vi "UDP Sender generic_2.vi"(1 "re-initialise":bool, 2 "Show panel":bool, 3 "Spots":T4[](array[typedef])=[{"Position"={"x"=6.0125e-05, "y"=5.4187499999999996e-05, "z"=7.0069138e-06}, "Intensity"=1.0, "Vortex Charge"=0, "Phase"=1.0, "NA Position"={"x"=0.0, "y"=0.0, "r"=1.0}, "Line Trapping"={"Vector"={"x"=0.0, "y"=0.0, "z"=0.0}, "Phase Gradient"=0.0}, "Amplitude Correction"=0.0}, {"Position"={"x"=5.4116381799999997e-05, "y"=3.98060334e-05, "z"=0.0}, "Intensity"=1.0, "Vortex Charge"=0, "Phase"=1.0, "NA Position"={"x"=0.0, "y"=0.0, "r"=1.0}, "Line Trapping"={"Vector"={"x"=0.0, "y"=0.0, "z"=0.0}, "Phase Gradient"=0.0}, "Amplitude Correction"=0.0}, {"Position"={"x"=7.662499999999999e-05, "y"=4.6e-05, "z"=0.0}, "Intensity"=1.0, "Vortex Charge"=0, "Phase"=1.0, "NA Position"={"x"=0.0, "y"=0.0, "r"=1.0}, "Line Trapping"={"Vector"={"x"=0.0, "y"=0.0, "z"=0.0}, "Phase Gradient"=0.0}, "Amplitude Correction"=0.0}] {"Amplitude Correction" step=0.1; "Line Trapping"."Phase Gradient" step=0.05; "Line Trapping"."Vector"."x" step=1e-06 format="%#_6p"; "Line Trapping"."Vector"."y" step=1e-06 format="%#_6p"; "Line Trapping"."Vector"."z" step=1e-06 format="%#_6p"; "NA Position"."r" step=1e-06; "NA Position"."y" step=1e-06; "NA Position"."x" step=1e-06; "Position"."z" step=1e-06; "Position"."y" step=1e-06; "Position"."x" step=1e-06; "Phase" step=0.7753; "Intensity" step=0.1}) -> (0 "length":i32=557)   [LabVIEW 2010]
doc: "This VI sends UDP packets to the hologram server so that it can display holograms. It also has a lot of settings on the front panel, which control most of the aspects of hologram generation and display.\n\n\n(the line below ensures settings are saved)\n[Red Tweezers Save Settings]"
uses:
  spot.ctl
  line_trapping.ctl
  red_tweezers_globals_INTERNAL.vi
  <vilib>/Analysis/7linalg.llb/Create Special Real Matrix.vi
  <vilib>/Analysis/baseanly.llb/Real A x B.vi
  <vilib>/Analysis/NI_AALPro.lvlib
  <vilib>/Analysis/NI_AALBase.lvlib
panel:
  in  "SLM Settings":T1(tab)=enum."Output Location"
  out "LUT":cluster{dbl, dbl}[](graph)=[{-3.141592653589793, 0.0}, {-2.938909256584, 0.0}, {-2.736225859578207, 0.0}, {-2.533542462572414, 0.0}, {-2.330859065566621, 0.0}, {-2.1281756685608277, 0.0}, {-1.9254922715550344, 0.0}, {-1.7228088745492414, 0.0}, {-1.5201254775434483, 0.0}, {-1.317442080537655, 0.0}, {-1.114758683531862, 0.013893883492187394}, {-0.9120752865260688, 0.08758036091961133}, {-0.7093918895202758, 0.17634603660070491}, {-0.5067084925144827, 0.2746032303815977}, {-0.3040250955086896, 0.37671834381730007}, {-0.10134169850289654, 0.4770577784628228}, {0.10134169850289654, 0.5700419053299409}, {0.30402509550868917, 0.6525515168106174}, {0.5067084925144831, 0.7248906022855592}, {0.7093918895202758, 0.7876162829469834}, {0.9120752865260693, 0.8412856799871068}, {1.1147586835318615, 0.8864559145981461}, {1.3174420805376554, 0.9236841079723185}, {1.5201254775434485, 0.9535273813018404}, {1.7228088745492416, 0.9765739527614036}, {1.9254922715550338, 0.993632504666451}, {2.1281756685608277, 1.0}, {2.330859065566621, 1.0}, {2.533542462572414, 1.0}, {2.736225859578207, 1.0}, {2.938909256584, 1.0}, {3.141592653589793, 1.0}]
  in  "LUT File":path=path "C:/Users/alinnenberger/Desktop/Cube/red_tweezers_1_4_rc0/slm2040.LUT"
  in  "Intensity Masking (0=off, 1=on, >1=partially on)":dbl
  in  "Full Screen":bool
  out "Monitor Picture":picture
  in  "Monitor":i32=1
  in  "Zernike Coefficients":dbl[](array[numeric])=[0.0, 20.0, 20.0, 0.0, 0.0, 0.0, 0.0, 0.0, 0.0, 0.0, 0.0, 0.0]
  in  "Enable":bool=TRUE
  in  "Multiplier":dbl=1.0
  out "Phase Map":dbl[][](graph)
  in  "Physical Geometry":T2={"Hologram Size"={"x"=0.0102, "y"=0.0102}, "Focal Length"=0.0045, "Wavelength"=1.064e-06} {"Hologram Size"."y" min=0.0 max=1.0 step=0.001 format="%#_3p"; "Hologram Size"."x" min=0.0 max=1.0 step=0.001 format="%#_3p"; "Focal Length" format="%#_3p"; "Wavelength" format="%#_6p"}
  in  "Zero Position On Camera/pixels":cluster{"X":dbl, "Y":dbl}={"X"=320.0, "Y"=240.0}
  in  "Camera Pixel Size/m":cluster{dbl, dbl}={1e-07, 1e-07} {"?" format="%#_4p"; "?" format="%#_4p"}
  in  "Illumination Centre (range: 0 to 1)":cluster{"x":dbl, "y":dbl}={"x"=0.5, "y"=0.5} {"y" min=0.0 max=1.0 step=0.001; "x" min=0.0 max=1.0 step=0.001}
  in  "Scale Spot Positions":cluster{"x":dbl, "y":dbl, "z":dbl}={"x"=1.0, "y"=1.0, "z"=1.0} {"z" step=0.05 format="%#_3p"; "y" step=0.05 format="%#_3p"; "x" step=0.05 format="%#_3p"}
  in  "Rotation (degrees)":dbl
  in  "Tab Control":T3(tab)
  out "message":string="<data>\n<uniform id=0>\n  3.000000\r\n</uniform>\n<uniform id=2>\n  60.125000 54.187500 7.006914 0.000000 1.000000 1.000000 0.000000 0.000000 0.000000 0.000000 1.000000 0.000000 0.000000 0.000000 0.000000 0.000000 54.116382 39.806033 0.000000 0.000000 1.000000 1.000000 0.000000 0.000000 0.000000 0.000000 1.000000 0.000000 0.000000 0.000000 0.000000 0.000000 76.625000 46.000000 0.000000 0.000000 1.000000 1.000000 0.000000 0.000000 0.000000 0.000000 1.000000 0.000000 0.000000 0.000000 0.000000 0.000000\r\n</uniform>\n<uniform id=1>\n  0.000000\r\n</uniform>\n</data>"
  in  "x":dbl[](array[numeric])=[0.0, 0.0, 0.0]
  in  "y":dbl[](array[numeric])=[0.0, 0.0, 0.0]
  in  "z":dbl[](array[numeric])=[0.0, 0.0, 0.0]
  in  "close":bool
  # "Look-Up Table\nThis curve controls the output level (0=black, 1=white) for a given phase on the SLM.  It can be used to optimise the hologram to direct as much light as possible into the first diffraction order, and is particularly useful when the SLM has a range of more or less than one wavelength."
  # "Intensity masking can modulate the LUT to shape intensity on the SLM.  Leave at 0 for most purposes."
  # "Find the SLM Monitor\nSelect the monitor that corresponds to the SLM.  Usually this will be the second monitor (i.e. number 2).  If you are using a BNS SLM, leave \"full screen\" unchecked; for Holoeye/Hamamatsu, push that button.\n\nThe box below shows the monitors attached to your computer, and a red box where the SLM window will appear.  The monitor numbers should be the same as those in the Windows monitor settings.  You can also click monitors below to select them."
  # "Aberration Correction\nThe engine allows Zernike polynomials to be added to the hologram to compensate for aberrations.  The coefficients can be adjusted here.  The polynomials included are the first 15, ignoring piston and tilt (as these are adjusted for each spot)."
  # "Scaling Factors\nYou should enter the dimensions of your system in the \"physical geometry\" box to set approximate scaling; the hologram size is the SLM size (normally square, as only the central square is used) AFTER any magnification when it's re-imaged, and the focal length is that of the objective lens.\n\nHere, you can also set the size of pixels on the camera (best done using a calibration slide) and the location of the zero order from the SLM.\n\nFine-tuning can be done on the \"Alignment & Centering\" tab."
  # "Centering\nIf the illumination of the SLM is off-centre, moving a spot in Z will also affect its position in X and Y (think of an off-centre lens).  The \"illumination centre\" can correct for this.  Setting this parameter correctly is particularly important if Laguerre-Gauss beams are to be used (i.e. spots with L not equal to 0).  The real centre of the hologram is at 0.5,0.5.  NB if this value is far from 0.5, 0.5 the system probably needs to be realigned."
  # "Scaling and Rotation\nThe scaling rand rotation controls allow you to compensate for the camera and SLM being rotated relative to each other, or for small variations from the geometrically predicted scale.  The scaling factors ought to be aroud unity.  Negative scaling factors will invert the corresponding axis.\nNB: Make sure the correct values are entered in the \"geometry\" tab first!"
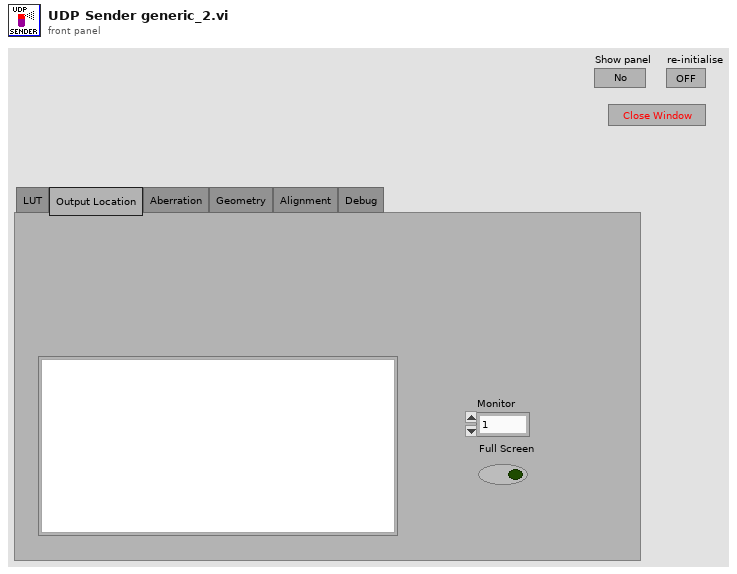
[diagram p1: front panel]
types:
  T1 = enum32{"LUT", "Output Location", "Aberration", "Geometry", "Alignment", "Debug"}
  T2 = cluster{"Hologram Size":cluster{"x":dbl, "y":dbl}, "Focal Length":dbl, "Wavelength":dbl}
  T3 = enum32{"Spots", "UDP Packets", "Field Tilt/Varying Astigmatism"}
  T4 = typedef "spot.ctl" = cluster{"Position":cluster{"x":dbl, "y":dbl, "z":dbl}, "Intensity":dbl, "Vortex Charge":i8, "Phase":dbl, "NA Position":cluster{"x":dbl, "y":dbl, "r":dbl}, "Line Trapping":T5, "Amplitude Correction":dbl}
  T5 = typedef "line_trapping.ctl" = cluster{"Vector":cluster{"x":dbl, "y":dbl, "z":dbl}, "Phase Gradient":dbl}
  T6 = enum32{"Identity", "Diagonal", "Toepliz", "Vandermonde", "Companion"}
  T7 = typedef "NI_Matrix.lvlib/RealMatrix.ctl" = dbl[][]
  T8 = typedef "LVMouseTypeDef.ctl" = cluster{"Mouse Position":cluster{"X":i32, "Y":i32}, "Mouse Modifiers":cluster{"Button Down":bool, "Shift Mod":bool, "Menu Mod":bool, "Option Mod":bool}}
  T9 = typedef "LVCursorListTypeDef.ctl" = cluster{"Name":string, "Color":u32, "Style":u8, "Point Style":u8, "Name Visible":bool, "Allow Drag":bool, "Cursor Mode":u32, "Plot":i32, "Index":i32, "Position":cluster{"X":dbl, "Y":dbl}, "X Scale":u32, "Y Scale":u32, "Watch Plots":i32[], "Watch All Plots":bool, "Plot Area":i32, "Label Offset":cluster{"X":dbl, "Y":dbl}}[]
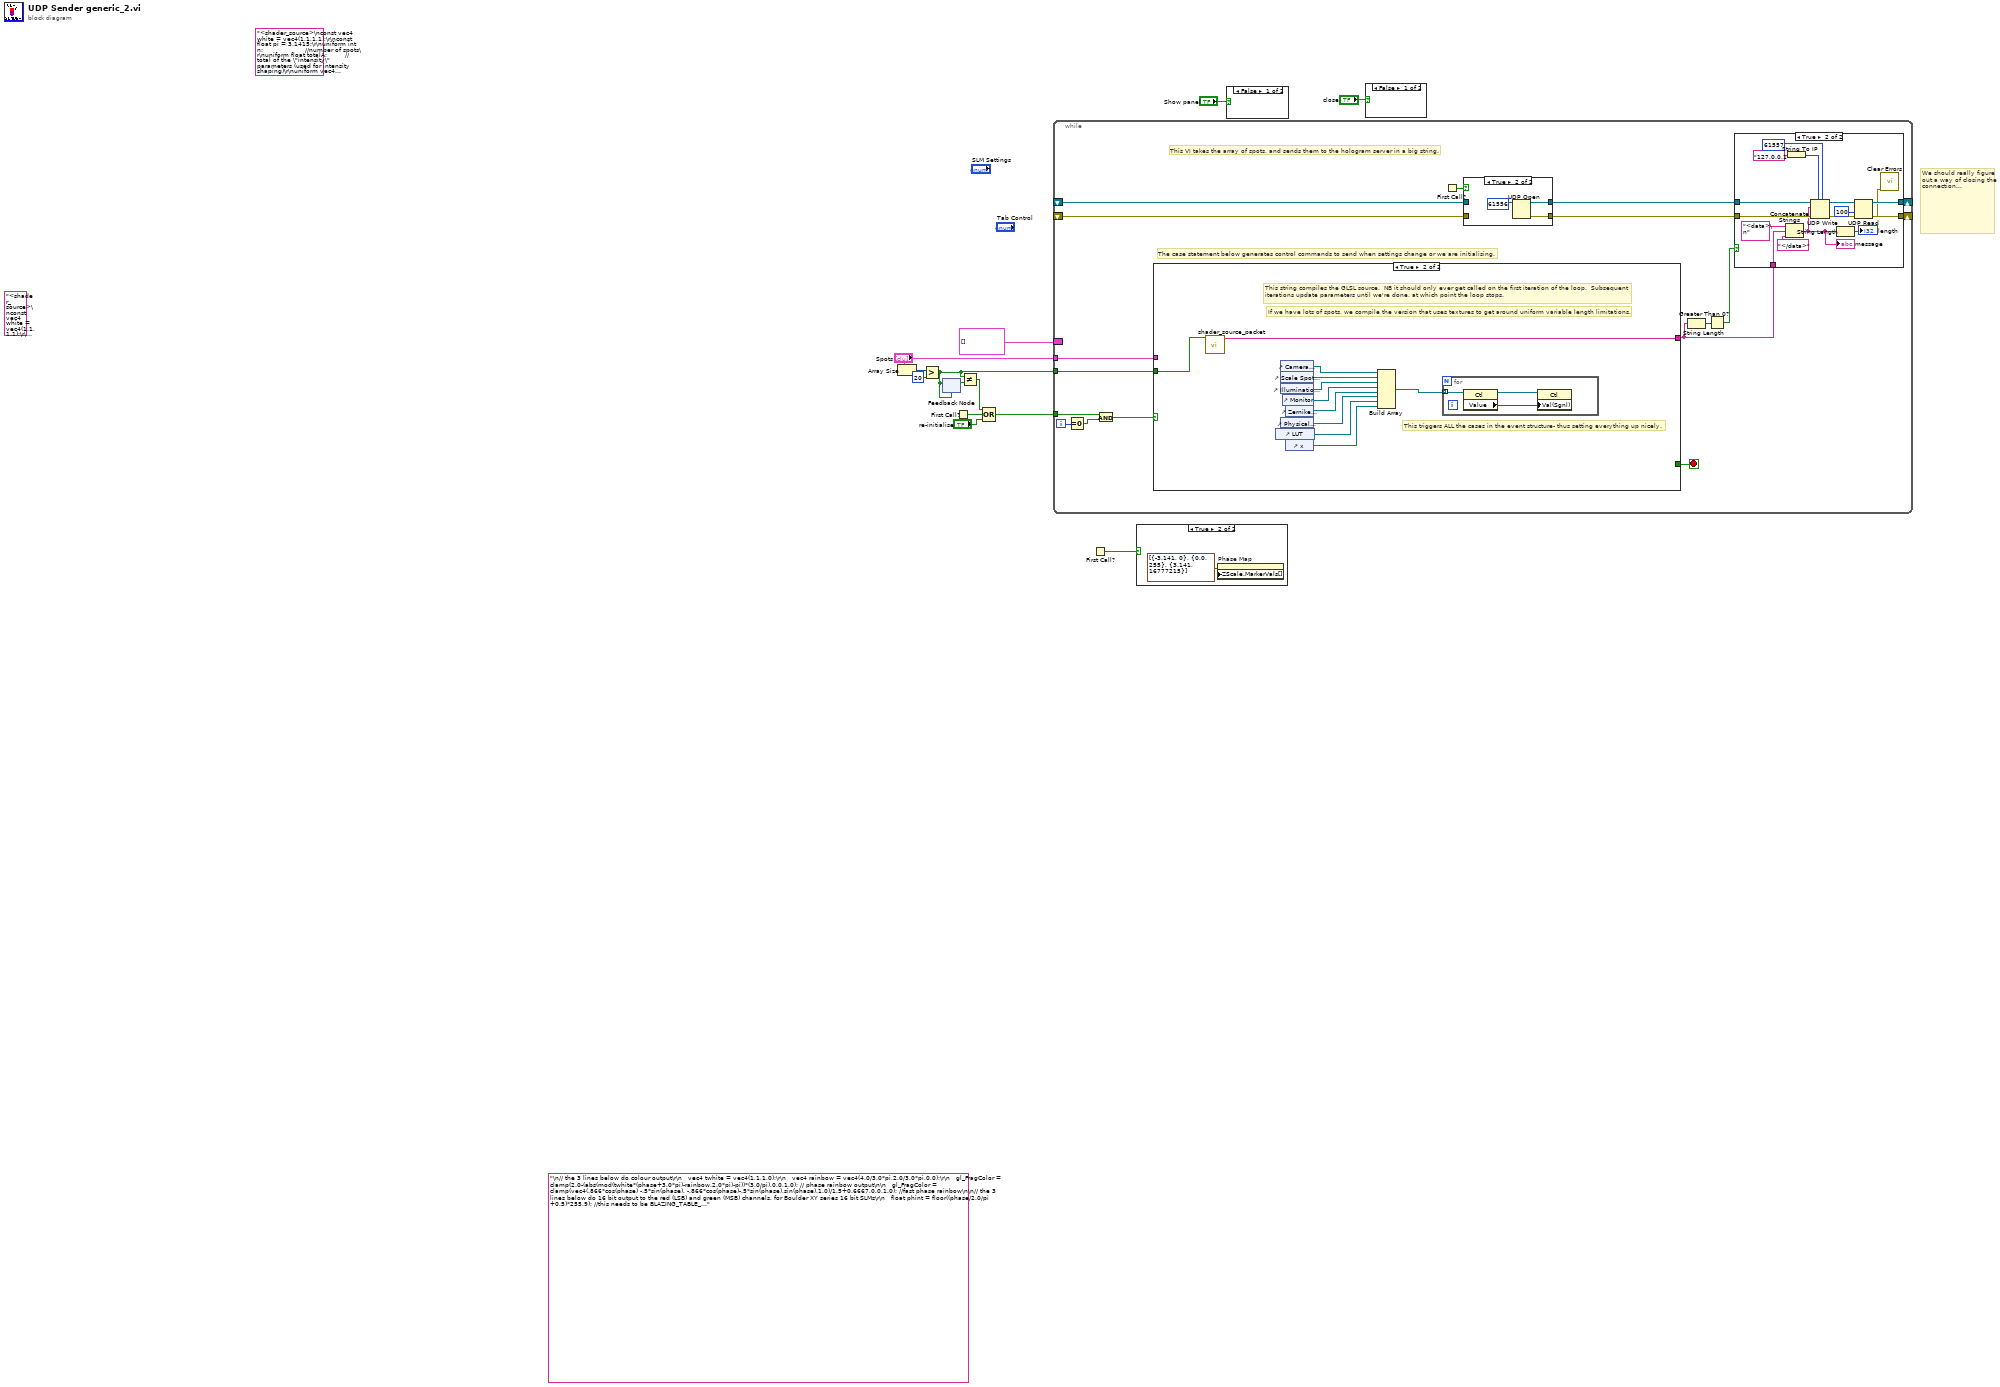
[diagram p0: block diagram]
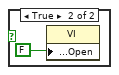
[diagram p3: hidden frame]
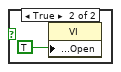
[diagram p4: hidden frame]
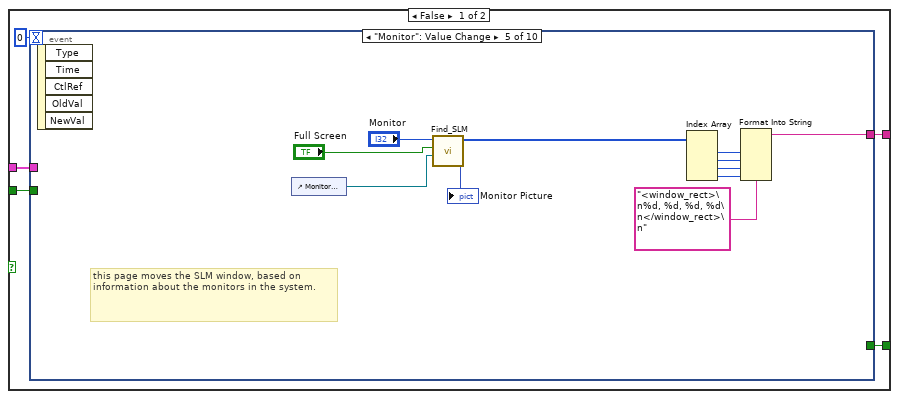
[diagram p6: hidden frame]
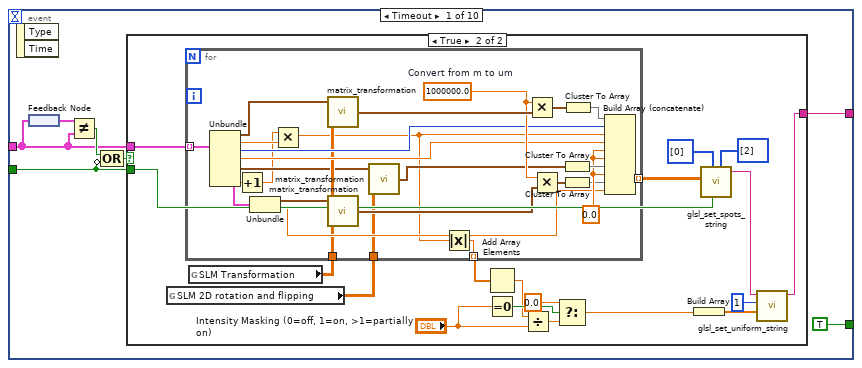
[diagram p7: hidden frame]
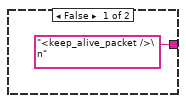
[diagram p8: hidden frame]
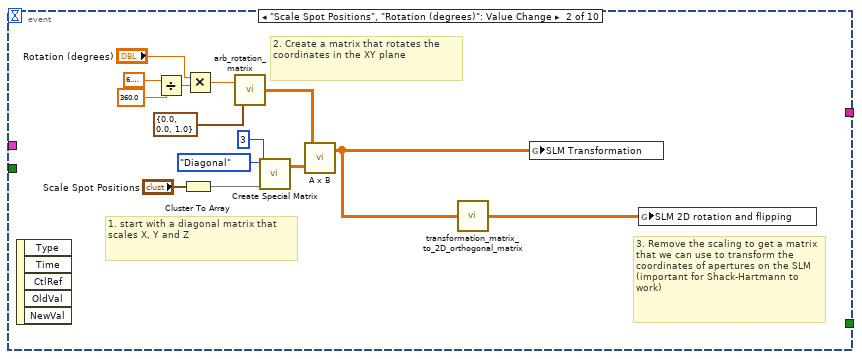
[diagram p9: hidden frame]
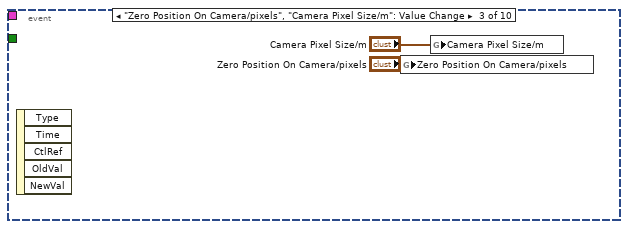
[diagram p10: hidden frame]
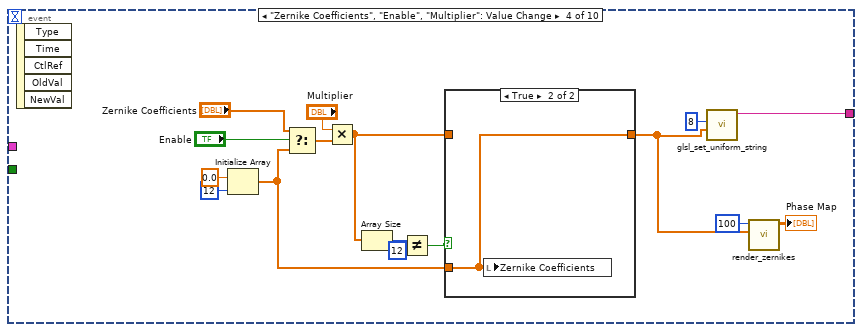
[diagram p11: hidden frame]
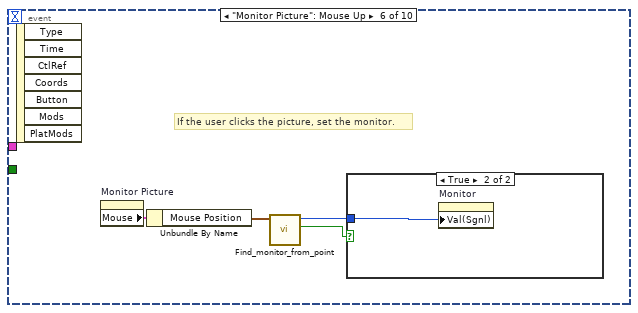
[diagram p13: hidden frame]
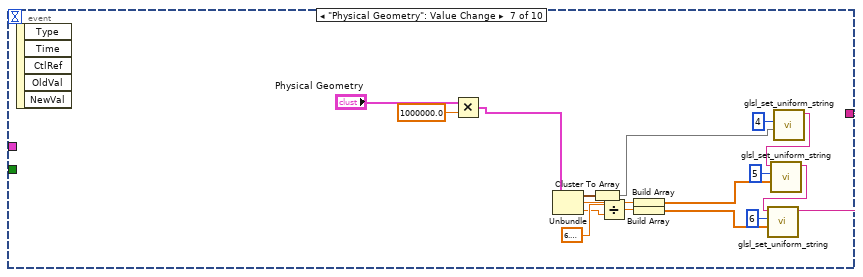
[diagram p15: hidden frame]
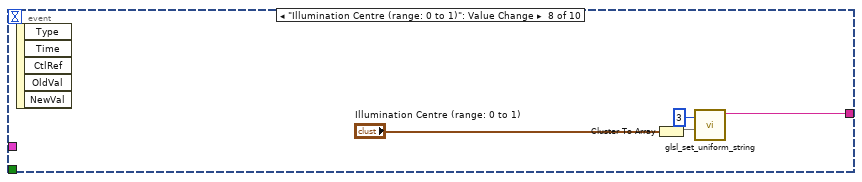
[diagram p16: hidden frame]
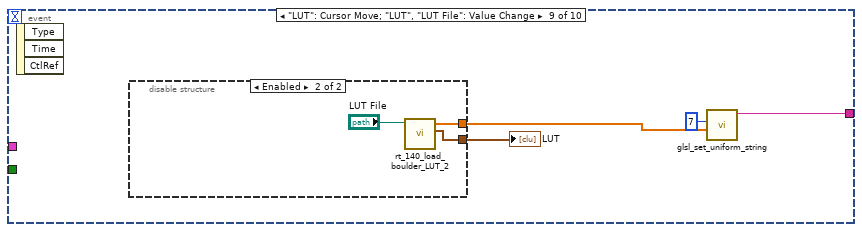
[diagram p17: hidden frame]
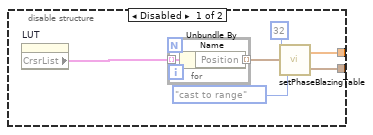
[diagram p18: hidden frame]
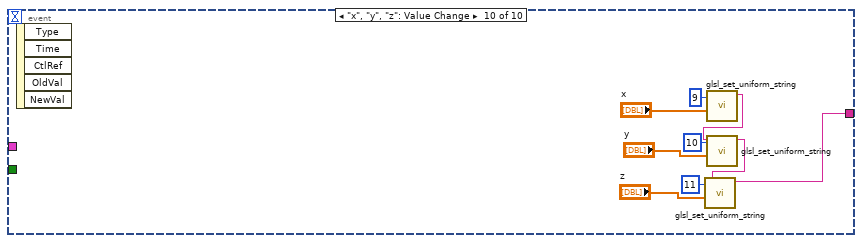
[diagram p19: hidden frame]
diagram:
  (unwired) "<shader_source>\nconst vec4 white = vec4(1,1,1,1);\r\nconst float pi = 3.1415;\r\nuniform int n;                     //number of spots\r\nuniform float totalA;         //total of the \"intensity\" parameters (used for intensity shaping)\r\nuniform sampler2D spots; //spot parameters- each spot corresponds to 4 vec4, first one is x,y,z,l, second one is amplitude, -,-,-\n\r                                            //element 0 x  y  z  l    (x,y,z in um and l is an integer)\n                                            //element 1 intensity (I) phase -  -\n                                            //element 2 na.x na.y na.r -  (the x, y position, and radius, of the spot on the SLM- useful for Shack-Hartmann holograms)\n                                            //element 3 line trapping x y z and phase gradient.  xyz define the size and angle of the line, phase gradient (between +/-1) is the\n                                            //scattering force component along the line.  Zero is usually a good choice for in-plane line traps\nuniform vec2 centre;        //=vec2(0.5,0.5);//centre of the hologram as a fraction of its size (usually 0.5,0.5)\r\nuniform vec2 size;            //=vec2(7000,7000);//size of the hologram in microns\r\nuniform float f;                 //=1600; //focal length in microns\r\nuniform float k;                //=9.36; //wavevector in 1/microns\r\nuniform float blazing[32]; //blazing function\r\nuniform vec4 zernikeCoefficients[3]; //zernike coefficients, matching the modes defined below\nuniform vec3 zernx;        //=vec3(0.0,0.0,0.0);\nuniform vec3 zerny;        //=vec3(0.0,0.0,0.0);\nuniform vec3 zernz;        //=vec3(0.0,0.0,0.0);\n\nvec4 spot(int i, int j){\n  return texture(spots, vec2( (float(j) +0.5) / 4.0, ( float(i) + 0.5) / float(n) ))*500.0 -250.0;\n}\n\nvoid main(void)\r\n{\n   float totalr=0.0;                                                //real and imaginary parts of the complex hologram for this pixel\r\n   float totali=0.0;\r\n   float phase;                                                       //phase of current pixel, due to the spot (in loop) or of the resultant hologram (after loop)\r\n   float amplitude;                                               //ditto for amplitude\r\n   vec2 xy=(gl_TexCoord[0].xy-centre)*size;    //current xy position in the hologram, in microns\r\n   float phi=atan(xy.x,xy.y);\t\t                              //angle of the line joining our point to the centre of the pattern\r\n   float length;                                                     //length of a line\r\n   vec4 pos=vec4(xy/f,1.0-dot(xy,xy)/2.0/f/f,phi/k);\r\n   vec4 na;                                                           //to be used later, inside the loop\r\n\t float sx;\r\n//Zernike polynomials\r\n   float x=xy.x/size.x*2.0;\n   float  y=xy.y/size.y*2.0; //x,y range from -1 to 1, because the Zernike modes want them to do that...\r\n   float r2=x*x+y*y;\r\n   vec4 zerna=vec4(2.0*x*y,2.0*r2-1.0,x*x-y*y,3.0*x*x*y-y*y*y); //zernike modes (2 -2, 2 0, 2 2, 3 -3)\r\n   vec4 zernb=vec4((3.0*r2-2.0)*y,(3.0*r2-2.0)*x,x*x*x-3.0*x*y*y,4.0*x*y*(x*x-y*y)); //3 -1 through 4 -4\r\n   vec4 zernc=vec4((4.0*r2-3.0)*zerna[0],6.0*r2*r2-6*r2+1,(4.0*r2-3.0)*zerna[2],x*x*x*x-6.0*x*x*y*y+y*y*y*y); //4 -2 through 4 4\r\n//probably want to redefine x,y,r2 if they are used below this line, but the are currently not.\n\n   vec4 varyingzernike=vec4(0.0,0.0,0.0,0.0);\n   varyingzernike.x=dot(zernx,zerna.xyz);\n   varyingzernike.y=dot(zerny,zerna.xyz);\n   varyingzernike.z=dot(zernz,zerna.xyz);\n\n   float j=0.0;                                                       //this loop goes through the spots and calculates the contribution from each one, summing\n                                                                            //real and imaginary parts as we go.\r\n   for(int i=0; i<n; i++){\n      amplitude=spot(i,1)[0];                             //amplitude of current spot\r\n      phase=k*dot(spot(i,0),pos)+spot(i,1)[1]; \n                                                                            //this is the basic gratings and lenses algorithm; phase=kx*x+ky*y+kz*(x^2+y^2)+l*theta\n\n      na = spot(i,2);                                           //restrict the spot to a region of the back aperture which is na[2] in radius, centred on na.xy\r\n      if(dot(na.xy-xy/size,na.xy-xy/size) > na[2]*na[2]){\n        amplitude = 0.0;\n      }\n//creates an xyz line trap, needs amplitude shaping.\n\r      vec4 line = spot(i,3);\n      length=sqrt(dot(line.xyz,line.xyz));\r\n      if(length>0.0){\r\n\t\t      sx=k*dot(vec4(pos.xyz,1.0*length),line);\r\n\t\t      if(sx!=0.0) amplitude*=sin(sx)/sx;\r\n      }\n\r                                                                 //finally, convert from amplitude+phase to real+imaginary for the summation\n      totalr += amplitude*sin(phase);\t  //the way atan is defined, we need to use sin for r and cos for i.\r\n      totali += amplitude*cos(phase);\r\n   }\n\r\n   amplitude = sqrt(totalr*totalr+totali*totali);\r\n   phase=atan(totalr,totali);\r\n   if(amplitude==0.0) phase=0.0;\r\n   if(totalA>0.0){ //do amplitude-shaping (dumps light into zero order when not needed)\r\n     phase *= clamp(amplitude/totalA,0.0,1.0);\r\n   }\r\n   phase += dot(zernikeCoefficients[0],zerna) + dot(zernikeCoefficients[1],zernb) + dot(zernikeCoefficients[2],zernc);\r\n   phase = mod(phase + pi, 2*pi) -pi;\n\r\n\n// the 3 lines below do blazed black and white output to all 3 colour channels (most SLMs use this)\n    //we split phase into two parts: phint is an integer between 0 and 30, alpha is a float between 0 and 0.99999999999999\n    //such that (phint + alpha)/31 maps onto 0...1.\n\r    //then we use the blazing array with linear interpolation to apply the LUT.\n\n   int phint = int(floor((phase/2.0/pi +0.5)*30.9999999)); //this needs to be BLAZING_TABLE_LENGTH-(something small)-1\r\n   float alpha = fract((phase/2.0/pi +0.5)*30.9999999);\r\n   gl_FragColor = white * blazing[phint]*(1.0-alpha)+blazing[phint+1]*alpha; //this uses the blazing table with linear interpolation\n\n//  gl_FragColor = spot(0,1);\n//  gl_FragColor = vec4(%%randcol%%);\n// gl_FragColor = gl_FragColor * vec4(%%randcol%%);\n//  gl_FragColor = texture(spots, gl_TexCoord[0].xy)*500.0-250.0;\n}\n</shader_source>\n\n<swap_buffers_at_refresh_rate>\n0\n</swap_buffers_at_refresh_rate>\n</data>"
  (unwired) "<shader_source>\nconst vec4 white = vec4(1,1,1,1);\r\nconst float pi = 3.1415;\r\nuniform int n;                     //number of spots\r\nuniform float totalA;         //total of the \"intensity\" parameters (used for intensity shaping)\r\nuniform vec4 spots[200]; //spot parameters- each spot corresponds to 4 vec4, first one is x,y,z,l, second one is amplitude, -,-,-\n\r                                            //element 0 x  y  z  l    (x,y,z in um and l is an integer)\n                                            //element 1 intensity (I) phase -  -\n                                            //element 2 na.x na.y na.r -  (the x, y position, and radius, of the spot on the SLM- useful for Shack-Hartmann holograms)\n                                            //element 3 line trapping x y z and phase gradient.  xyz define the size and angle of the line, phase gradient (between +/-1) is the\n                                            //scattering force component along the line.  Zero is usually a good choice for in-plane line traps\nuniform vec2 centre;        //=vec2(0.5,0.5);//centre of the hologram as a fraction of its size (usually 0.5,0.5)\r\nuniform vec2 size;            //=vec2(7000,7000);//size of the hologram in microns\r\nuniform float f;                 //=1600; //focal length in microns\r\nuniform float k;                //=9.36; //wavevector in 1/microns\r\nuniform float blazing[32]; //blazing function\r\nuniform vec4 zernikeCoefficients[3]; //zernike coefficients, matching the modes defined below\nuniform vec3 zernx;        //=vec3(0.0,0.0,0.0);\nuniform vec3 zerny;        //=vec3(0.0,0.0,0.0);\nuniform vec3 zernz;        //=vec3(0.0,0.0,0.0);\n\nvec4 spot(int i, int j){\n//  return texture(spots, vec2( (float(j) +0.5) / 4.0, ( float(i) + 0.5) / float(n) ))*500.0 -250.0;\n  return spots[4*i +j];\n}\n\nvoid main(void)\r\n{\n   float totalr=0.0;                                                //real and imaginary parts of the complex hologram for this pixel\r\n   float totali=0.0;\r\n   float phase;                                                       //phase of current pixel, due to the spot (in loop) or of the resultant hologram (after loop)\r\n   float amplitude;                                               //ditto for amplitude\r\n   vec2 xy=(gl_TexCoord[0].xy-centre)*size;    //current xy position in the hologram, in microns\r\n   float phi=atan(xy.x,xy.y);\t\t                              //angle of the line joining our point to the centre of the pattern\r\n   float length;                                                     //length of a line\r\n   vec4 pos=vec4(xy/f,1.0-dot(xy,xy)/2.0/f/f,phi/k);\r\n   vec4 na;                                                           //to be used later, inside the loop\r\n\t float sx;\r\n//Zernike polynomials\r\n   float x=xy.x/size.x*2.0;\n   float  y=xy.y/size.y*2.0; //x,y range from -1 to 1, because the Zernike modes want them to do that...\r\n   float r2=x*x+y*y;\r\n   vec4 zerna=vec4(2.0*x*y,2.0*r2-1.0,x*x-y*y,3.0*x*x*y-y*y*y); //zernike modes (2 -2, 2 0, 2 2, 3 -3)\r\n   vec4 zernb=vec4((3.0*r2-2.0)*y,(3.0*r2-2.0)*x,x*x*x-3.0*x*y*y,4.0*x*y*(x*x-y*y)); //3 -1 through 4 -4\r\n   vec4 zernc=vec4((4.0*r2-3.0)*zerna[0],6.0*r2*r2-6*r2+1,(4.0*r2-3.0)*zerna[2],x*x*x*x-6.0*x*x*y*y+y*y*y*y); //4 -2 through 4 4\r\n//probably want to redefine x,y,r2 if they are used below this line, but the are currently not.\n\n   vec4 varyingzernike=vec4(0.0,0.0,0.0,0.0);\n   varyingzernike.x=dot(zernx,zerna.xyz);\n   varyingzernike.y=dot(zerny,zerna.xyz);\n   varyingzernike.z=dot(zernz,zerna.xyz);\n\n   float j=0.0;                                                       //this loop goes through the spots and calculates the contribution from each one, summing\n                                                                            //real and imaginary parts as we go.\r\n   for(int i=0; i<n; i++){\n      amplitude=spot(i,1)[0];                             //amplitude of current spot\r\n      phase=k*dot(spot(i,0),pos)+spot(i,1)[1]; \n                                                                            //this is the basic gratings and lenses algorithm; phase=kx*x+ky*y+kz*(x^2+y^2)+l*theta\n\n      na = spot(i,2);                                           //restrict the spot to a region of the back aperture which is na[2] in radius, centred on na.xy\r\n      if(dot(na.xy-xy/size,na.xy-xy/size) > na[2]*na[2]){\n        amplitude = 0.0;\n      }\n//creates an xyz line trap, needs amplitude shaping.\n\r      vec4 line = spot(i,3);\n      length=sqrt(dot(line.xyz,line.xyz));\r\n      if(length>0.0){\r\n\t\t      sx=k*dot(vec4(pos.xyz,1.0*length),line);\r\n\t\t      if(sx!=0.0) amplitude*=sin(sx)/sx;\r\n      }\n\r                                                                 //finally, convert from amplitude+phase to real+imaginary for the summation\n      totalr += amplitude*sin(phase);\t  //the way atan is defined, we need to use sin for r and cos for i.\r\n      totali += amplitude*cos(phase);\r\n   }\n\r\n   amplitude = sqrt(totalr*totalr+totali*totali);\r\n   phase=atan(totalr,totali);\r\n   if(amplitude==0.0) phase=0.0;\r\n   if(totalA>0.0){ //do amplitude-shaping (dumps light into zero order when not needed)\r\n     phase *= clamp(amplitude/totalA,0.0,1.0);\r\n   }\r\n   phase += dot(zernikeCoefficients[0],zerna) + dot(zernikeCoefficients[1],zernb) + dot(zernikeCoefficients[2],zernc);\r\n   phase = mod(phase + pi, 2*pi) -pi;\n\r\n\n// the 3 lines below do blazed black and white output to all 3 colour channels (most SLMs use this)\n    //we split phase into two parts: phint is an integer between 0 and 30, alpha is a float between 0 and 0.99999999999999\n    //such that (phint + alpha)/31 maps onto 0...1.\n\r    //then we use the blazing array with linear interpolation to apply the LUT.\n\n   int phint = int(floor((phase/2.0/pi +0.5)*30.9999999)); //this needs to be BLAZING_TABLE_LENGTH-(something small)-1\r\n   float alpha = fract((phase/2.0/pi +0.5)*30.9999999);\r\n   gl_FragColor = white * blazing[phint]*(1.0-alpha)+blazing[phint+1]*alpha; //this uses the blazing table with linear interpolation\n\n//  gl_FragColor = spot(0,1);\n//  gl_FragColor = vec4(%%randcol%%);\n// gl_FragColor = gl_FragColor * vec4(%%randcol%%);\n//  gl_FragColor = texture(spots, gl_TexCoord[0].xy)*500.0-250.0;\n}\n</shader_source>\n\n<swap_buffers_at_refresh_rate>\n0\n</swap_buffers_at_refresh_rate>\n</data>"
  (unwired) "\n// the 3 lines below do colour output\r\n   vec4 twhite = vec4(1,1,1,0);\r\n   vec4 rainbow = vec4(4.0/3.0*pi,2.0/3.0*pi,0,0);\r\n   gl_FragColor = clamp(2.0-(abs(mod(twhite*(phase+3.0*pi)-rainbow,2.0*pi)-pi))*(3.0/pi),0.0,1.0); // phase rainbow output\n\n   gl_FragColor = clamp(vec4(.866*cos(phase) -.5*sin(phase), -.866*cos(phase)-.5*sin(phase),sin(phase),1.0)/1.5+0.6667,0.0,1.0); //fast phase rainbow\n\n// the 3 lines below do 16 bit output to the red (LSB) and green (MSB) channels, for Boulder XY series 16 bit SLMs\r\n   float phint = floor((phase/2.0/pi +0.5)*255.9); //this needs to be BLAZING_TABLE_LENGTH-(something small)\r\n   float alpha = fract((phase/2.0/pi +0.5)*255.9);\r\n   gl_FragColor = vec4(alpha,phint/255.0,0.0,1.0); //this uses the blazing table with linear interpolation\r\n\n// This one does grayscale output, black=-pi white=pi\r\n   gl_FragColor = white*(phase/2.0/pi +0.5);\n\r\n// the 3 lines below do blazed black and white output to all 3 colour channels (most SLMs use this)\r\n   int phint = int(floor((phase/2.0/pi +0.5)*30.9999999)); //this needs to be BLAZING_TABLE_LENGTH-(something small)-1\r\n   float alpha = fract((phase/2.0/pi +0.5)*30.9999999);\r\n   gl_FragColor = white * blazing[phint]*(1.0-alpha)+blazing[phint+1]*alpha; //this uses the blazing table with linear interpolation\n\n// \t gl_FragColor = float(n)*spots[0][1]/4.0*white;\r\n// \t gl_FragColor = mod(y*5,1.0)*white;\n//   gl_FragColor = white*blazing[16];\n\r"
  # "We should really figure out a way of closing the connection..."
  n1 = Array Size(array="Spots") -> (size(s)=w6:i32)
  n2 = Greater?(x=w6, y=20) -> (0:w2:bool)
  n3 = feedback #1(w2) -> (w8:bool)
  n4 = feedback-in #1(w2) -> ()
  n5 = First Call?() -> (First Call?: T/F=w5:bool)
  n6 = Not Equal?(x=w2, y=w8) -> (x != y?=w9:bool)
  n7 = Compound Arithmetic op=OR(w9, w5, "re-initialise") -> (w4:bool)
  n8 = while {
    shift-right: [w29] -> _
    shift-left: _ -> [w28]
    shift-right: [w30] -> _
    shift-left: _ -> [w27]
    border: T4[] [] ("Spots 2") -> [_]
    tunnel: w4 -> [w19]
    tunnel: w2 -> [w18]
    tunnel: "Spots" -> [w14]
    i -> [w16]
    stop <- w23 stop-if-true
    # "The case statement below generates control commands to send when settings change or we are initialising."
    # "This VI takes the array of spots, and sends them to the hologram server in a big string."
    n9 = Equal To 0?(x=w16) -> (x = 0?=w15:bool)
    n10 = And(x=w19, y=w15) -> (x .and. y?=w17:bool)
    n11 = case shown="True" w17 {
      tunnel: [w51 w201] -> w22
      tunnel: [w50 _] -> w23
      tunnel: w14 -> [w49 _]
      tunnel: w18 -> [w48 w200]
      frame False {
        n12 = event shown="[4] \"Monitor\": Value Change" {
          selector: _ -> [_ _ _ _ _ _ _ _ _ _]
          dyn-events: _ -> [_ _ _ _ _ _ _ _ _ _]
          timeout: 0 -> [_ _ _ _ _ _ _ _ _ _]
          tunnel: [w59 _ _ w121 w140 _ w155 w172 w176 w191] -> w51
          tunnel: [TRUE _ _ _ _ _ _ _ _ _] -> w50
          tunnel: w49 -> [w55 _ _ _ _ _ _ _ _ _]
          tunnel: w48 -> [w54 _ _ _ _ _ _ _ _ _]
          event Timeout {
            n13 = event-data() -> ()  [unwired: 1 in, 2 out]
            n14 = feedback #2() -> (w56:T4[])
            n15 = feedback-in #2(w55) -> ()
            n16 = Not Equal?(x=w56, y=w55) -> (x != y?=w57:bool)
            n17 = Compound Arithmetic op=OR(w57, invert w54) -> (w53:bool)
            n18 = case shown="True" w53 {
              tunnel: ["<keep_alive_packet />\n" ("Uniform-setting string") w69] -> w59
              tunnel: w55 -> [_ w62]
              tunnel: w54 -> [_ w61]
              frame False {
              }
              frame True {
                n19 = global read "red_tweezers_globals_INTERNAL.vi" "SLM 2D rotation and flipping"() -> (w67:T7)
                n20 = global read "red_tweezers_globals_INTERNAL.vi" "SLM Transformation"() -> (w68:T7)
                n21 = for {
                  tunnel: w62 -> [w102] mode=indexing
                  tunnel: [w99] -> w70 mode=indexing
                  tunnel: [w95] -> w66 mode=indexing
                  tunnel: w68 -> [w86]
                  tunnel: w67 -> [w82]
                  w91 = 0.0 ("element")
                  w96 = 1000000.0  # Convert from m to um
                  n22 = Unbundle(w102) -> ("Position"=w87:cluster{"x":dbl, "y":dbl, "z":dbl}, "Intensity"=w93:dbl, "Vortex Charge"=w94:i8, "Phase"=w92:dbl, "NA Position"=w84:cluster{"x":dbl, "y":dbl, "r":dbl}, "Line Trapping"=w100:T5, "Amplitude Correction"=w80:dbl)
                  n23 = Increment(x=w80) -> (x+1=w79:dbl)
                  n24 = Unbundle(w100) -> ("Vector"=w88:cluster{"x":dbl, "y":dbl, "z":dbl}, "Phase Gradient"=w89:dbl)
                  n25 = Multiply(x=w79, y=w93) -> (x*y=w81:dbl)
                  n26 = call "matrix_transformation.vi"("Transformation Matrix"=w86, "Input Vector"=w87) -> ("Output Vector"=w104:cluster{dbl, dbl, dbl})  [unwired: 1 in, 1 out]
                  n27 = call "matrix_transformation.vi"("Transformation Matrix"=w86, "Input Vector"=w88) -> ("Output Vector"=w85:cluster{dbl, dbl, dbl})  [unwired: 1 in, 1 out]
                  n28 = call "matrix_transformation.vi"("Transformation Matrix"=w82, "Input Vector"=w84) -> ("Output Vector"=w83:cluster{dbl, dbl, dbl})  [unwired: 1 in, 1 out]
                  n29 = Absolute Value(x=w81) -> (abs(x)=w99:dbl)
                  n30 = Multiply(x=w96, y=w104) -> (x*y=w98:cluster{dbl, dbl, dbl})
                  n31 = Multiply(x=w96, y=w85) -> (x*y=w97:cluster{dbl, dbl, dbl})
                  n32 = Cluster To Array(cluster=w83) -> (array=w101:dbl[])
                  n33 = Cluster To Array(cluster=w97) -> (array=w90:dbl[])
                  n34 = Cluster To Array(cluster=w98) -> (array=w103:dbl[])
                  n35 = Build Array (concatenate)(w103, w94, w81, w92, w91, w91, w101, w91, w90, w89) -> (w95:dbl[])
                }
                n36 = Add Array Elements(numeric array=w70) -> (sum=w71:dbl)
                n37 = Equal To 0?(x="Intensity Masking (0=off, 1=on, >1=partially on)") -> (x = 0?=w74:bool)
                n38 = Divide(x=w71, y="Intensity Masking (0=off, 1=on, >1=partially on)") -> (x/y=w73:dbl)
                n39 = Select(t=0.0, s=w74, f=w73) -> (s? t:f=w77:dbl)
                n40 = Build Array(w77) -> (w78:dbl[])
                n41 = call "glsl_set_spots_string.vi"("spots uniforms"=i32[] [2], "Use Textures?"=w61, "n uniforms"=i32[] [0], "Spots (2D Array)"=w66) -> ("Uniform-Setting String"=w65:string)  [unwired: 7 in]
                n42 = call "glsl_set_uniform_string.vi"("Uniform Value"=w78, "uniform index"=1, "initial string"=w65) -> ("Uniform-setting string"=w69:string)  [unwired: 3 in, 1 out]
              }
            }
          }
          event "Scale Spot Positions", "Rotation (degrees)": Value Change {
            # "3. Remove the scaling to get a matrix that we can use to transform the coordinates of apertures on the SLM (important for Shack-Hartmann to work)"
            # "2. Create a matrix that rotates the coordinates in the XY plane"
            # "1. start with a diagonal matrix that scales X, Y and Z"
            n43 = event-data() -> ()  [unwired: 1 in, 5 out]
            n44 = Divide(x=6.283185307179586, y=360.0) -> (x/y=w110:dbl)
            n45 = Cluster To Array(cluster="Scale Spot Positions") -> (array=w115:dbl[])
            n46 = Multiply(x="Rotation (degrees)", y=w110) -> (x*y=w108:dbl)
            n47 = call "arb_rotation_matrix.vi"("Unit Vector"=cluster{dbl, dbl, dbl} {0.0, 0.0, 1.0}, "theta"=w108) -> ("Real Matrix"=w113:T7)
            n48 = call-poly <vilib>:"Create Special Matrix.vi"("matrix type"=T6."Diagonal", "matrix size"=3, "Input Vector1"=w115) -> ("Special Matrix"=w112:T7)  [unwired: 2 in, 1 out]
            n49 = call-poly <vilib>:"A x B.vi"("B"=w112, "A"=w113) -> ("A x B"=w106:T7)  [unwired: 1 out]
            n50 = call "transformation_matrix_to_2D_orthogonal_matrix.vi"("A x B"=w106) -> ("Real Matrix"=w105:T7)
            n51 = global write "red_tweezers_globals_INTERNAL.vi" "SLM Transformation"(w106) -> ()
            n52 = global write "red_tweezers_globals_INTERNAL.vi" "SLM 2D rotation and flipping"(w105) -> ()
          }
          event "Zero Position On Camera/pixels", "Camera Pixel Size/m": Value Change {
            n53 = event-data() -> ()  [unwired: 1 in, 5 out]
            n54 = global write "red_tweezers_globals_INTERNAL.vi" "Zero Position On Camera/pixels"("Zero Position On Camera/pixels") -> ()
            n55 = global write "red_tweezers_globals_INTERNAL.vi" "Camera Pixel Size/m"("Camera Pixel Size/m") -> ()
          }
          event "Zernike Coefficients", "Enable", "Multiplier": Value Change {
            n56 = event-data() -> ()  [unwired: 1 in, 5 out]
            n57 = Initialize Array(0.0 ("element"), 12 ("dimension size")) -> (w124:dbl[])
            n58 = Select(t="Zernike Coefficients", s="Enable", f=w124) -> (s? t:f=w131:dbl[])
            n59 = Multiply(x="Multiplier", y=w131) -> (x*y=w123:dbl[])
            n60 = Array Size(array=w123) -> (size(s)=w127:i32)
            n61 = Not Equal?(x=w127, y=12) -> (x != y?=w125:bool)
            n62 = case shown="True" w125 {
              tunnel: w124 -> [_ w138]
              tunnel: w123 -> [w137 _]
              tunnel: [w137 w138] -> w122
              frame False {
              }
              frame True {
                n63 = local write "Zernike Coefficients"(w138) -> ()
              }
            }
            n64 = call "glsl_set_uniform_string.vi"("Uniform Value"=w122, "uniform index"=8) -> ("Uniform-setting string"=w121:string)  [unwired: 4 in, 1 out]
            n65 = call "render_zernikes.vi"("Size"=100, "Coefficients"=w122) -> ("Phase Map"=→"Phase Map":dbl[][])  [unwired: 6 out]
          }
          event "Monitor": Value Change {
            # "this page moves the SLM window, based on information about the monitors in the system."
            n66 = event-data() -> ()  [unwired: 1 in, 5 out]
            n67 = control-ref of="Monitor Picture"() -> (w147:refnum<vi>)
            n68 = call "Find_SLM.vi"("Picture Control"=w147, "Full Screen"="Full Screen", "Monitor"="Monitor") -> ("Monitor Picture"=→"Monitor Picture":picture, "Window Rect"=w141:i16[])  [unwired: 5 in, 2 out]
            n69 = Index Array(array=w141) -> (element #1=w143:i16, element #2=w144:i16, element #3=w145:i16, element #4=w146:i16)  [unwired: 4 in]
            n70 = Format Into String(format string="<window_rect>\n%d, %d, %d, %d\n</window_rect>\n", w143, w144, w145, w146) -> (resulting string=w140:string)  [unwired: 2 in, 1 out]
          }
          event "Monitor Picture": Mouse Up {
            # "If the user clicks the picture, set the monitor."
            n71 = event-data() -> ()  [unwired: 1 in, 7 out]
            n72 = property on="Monitor Picture" class="Pict"() -> ("Mouse"=w153:T8)  [unwired: 2 in, 2 out]
            n73 = Unbundle By Name(w153) -> ("Mouse Position"=w152:cluster{"X":i32, "Y":i32})
            n74 = call "Find_monitor_from_point.vi"("Point"=w152) -> ("In Monitor"=w151:bool, "Monitor"=w150:i32)  [unwired: 9 in]
            n75 = case shown="True" w151 {
              tunnel: w150 -> [_ w154]
              frame False {
              }
              frame True {
                n76 = property on="Monitor" class="DigNum (strict)"("Val(Sgnl)"=w154) -> ()  [unwired: 2 in, 2 out]
              }
            }
          }
          event "Physical Geometry": Value Change {
            n77 = event-data() -> ()  [unwired: 1 in, 5 out]
            n78 = Multiply(x="Physical Geometry", y=1000000.0 ("Wavevector (2pi/wavelength)")) -> (x*y=w163:T2)
            n79 = Unbundle(w163) -> ("Hologram Size"=w164:cluster{"x":dbl, "y":dbl}, "Focal Length"=w167:dbl, "Wavelength"=w170:dbl)
            n80 = Cluster To Array(cluster=w164) -> (array=w165:dbl[])
            n81 = Divide(x=6.283185307179586, y=w170) -> (x/y=w169:dbl)
            n82 = Build Array(w167) -> (w166:dbl[])
            n83 = Build Array(w169) -> (w168:dbl[])
            n84 = call "glsl_set_uniform_string.vi"("Uniform Value"=w165, "uniform index"=4) -> ("Uniform-setting string"=w157:string)  [unwired: 4 in, 1 out]
            n85 = call "glsl_set_uniform_string.vi"("Uniform Value"=w166, "uniform index"=5, "initial string"=w157) -> ("Uniform-setting string"=w156:string)  [unwired: 3 in, 1 out]
            n86 = call "glsl_set_uniform_string.vi"("Uniform Value"=w168, "uniform index"=6, "initial string"=w156) -> ("Uniform-setting string"=w155:string)  [unwired: 3 in, 1 out]
          }
          event "Illumination Centre (range: 0 to 1)": Value Change {
            n87 = event-data() -> ()  [unwired: 1 in, 5 out]
            n88 = Cluster To Array(cluster="Illumination Centre (range: 0 to 1)") -> (array=w174:dbl[])
            n89 = call "glsl_set_uniform_string.vi"("Uniform Value"=w174, "uniform index"=3) -> ("Uniform-setting string"=w172:string)  [unwired: 4 in, 1 out]
          }
          event "LUT": Cursor Move; "LUT", "LUT File": Value Change {
            n90 = event-data() -> ()  [unwired: 1 in, 3 out]
            n91 = disable-structure shown="Enabled" {
              disable-tunnel: [w185 w190] -> w178
              disable-tunnel: [w181 w189] -> w177
              frame Disabled {
                n92 = property on="LUT" class="XYGraph (strict)"() -> ("CrsrList"=w180:T9)  [unwired: 2 in, 2 out]
                n93 = for {
                  tunnel: w180 -> [w187] mode=indexing
                  tunnel: [w186] -> w184 mode=indexing
                  n94 = Unbundle By Name(w187) -> ("Position"=w186:cluster{"X":dbl, "Y":dbl})
                }
                n95 = call "setPhaseBlazingTable.vi"("-¹..¹ range control"=enum16{"wrap round", "cast to range"}."cast to range", "Anchor Points"=w184, "#elements (default 256)"=32) -> ("blazing graph"=w181:cluster{dbl, dbl}[], "blazing table"=w185:dbl[])
              }
              frame Enabled {
                n96 = call "rt_140_load_boulder_LUT_2.vi"("LUT File"="LUT File") -> ("'blazing function'"=w189:cluster{"X":dbl, "Y":dbl}[], "blazing table"=w190:dbl[])  [unwired: 8 in, 1 out]
              }
            }
            "LUT" <- w177
            n97 = call "glsl_set_uniform_string.vi"("Uniform Value"=w178, "uniform index"=7) -> ("Uniform-setting string"=w176:string)  [unwired: 4 in, 1 out]
          }
          event "x", "y", "z": Value Change {
            n98 = event-data() -> ()  [unwired: 1 in, 5 out]
            n99 = call "glsl_set_uniform_string.vi"("Uniform Value"="x", "uniform index"=9) -> ("Uniform-setting string"=w195:string)  [unwired: 4 in, 1 out]
            n100 = call "glsl_set_uniform_string.vi"("Uniform Value"="y", "uniform index"=10, "initial string"=w195) -> ("Uniform-setting string"=w196:string)  [unwired: 3 in, 1 out]
            n101 = call "glsl_set_uniform_string.vi"("Uniform Value"="z", "uniform index"=11, "initial string"=w196) -> ("Uniform-setting string"=w191:string)  [unwired: 3 in, 1 out]
          }
        }
      }
      frame True {
        # "If we have lots of spots, we compile the version that uses textures to get around uniform variable length limitations."
        # "This string compiles the GLSL source.  NB it should only ever get called on the first iteration of the loop.  Subsequent iterations update parameters until we're done, at which point the loop stops."
        # "This triggers ALL the cases in the event structure- thus setting everything up nicely."
        n102 = call "shader_source_packet.vi"(">50 Spots"=w200) -> ("Shader Source,"=w201:string)  [unwired: 9 in]
        n103 = control-ref of="LUT"() -> (w207:refnum<vi>)
        n104 = control-ref of="Camera Pixel Size/m"() -> (w202:refnum<vi>)
        n105 = control-ref of="Scale Spot Positions"() -> (w204:refnum<vi>)
        n106 = control-ref of="Illumination Centre (range: 0 to 1)"() -> (w210:refnum<vi>)
        n107 = control-ref of="Physical Geometry"() -> (w208:refnum<vi>)
        n108 = control-ref of="Monitor"() -> (w203:refnum<vi>)
        n109 = control-ref of="Zernike Coefficients"() -> (w209:refnum<vi>)
        n110 = control-ref of="x"() -> (w206:refnum<vi>)
        n111 = Build Array(w202, w204, w210, w203, w209, w208, w207, w206) -> (w205:refnum<vi>[])
        n112 = for {
          tunnel: w205 -> [w213] mode=indexing
          n113 = property class="Ctl"(reference=w213) -> (reference out=w211:refnum<vi>, "Value"=w212:variant)  [unwired: 1 in, 1 out]
          n114 = property class="Ctl"(reference=w211, "Val(Sgnl)"=w212) -> ()  [unwired: 1 in, 2 out]
        }
      }
    }
    n115 = First Call?() -> (First Call?: T/F=w24:bool)
    n116 = case shown="True" w24 {
      tunnel: [w215 w217] -> w26
      tunnel: [w214 w216] -> w25
      tunnel: w28 -> [w215 _]
      tunnel: w27 -> [w214 _]
      frame False {
      }
      frame True {
        n117 = UDP Open(11:u16 61556 ("Local Port")) -> (port=w217:refnum<k16>, 0:w216:errorcluster)  [unwired: 1 in, 4 out]
      }
    }
    n118 = String Length(string=w22) -> (length=w21:i32)
    n119 = Greater Than 0?(x=w21) -> (x > 0?=w20:bool)
    n120 = case shown="True" w20 {
      tunnel: [w31 w46] -> w30
      tunnel: [w32 w35] -> w29
      tunnel: w26 -> [w32 w44]
      tunnel: w25 -> [w31 w42]
      tunnel: w22 -> [_ w36]
      frame False {
      }
      frame True {
        n121 = Concatenate Strings("<data>\n" ("Data String"), w36, "</data>" ("Data String")) -> (w40:string)
        "message" <- w40
        n122 = String To IP(1:"127.0.0.1" ("Remote Host")) -> (0:w38:u32)
        n123 = UDP Write(address=w38, port or service name=u16 61557 ("Remote Port"), connection ID=w44, data in=w40, 8:w42) -> (error out=w46:errorcluster, 3:w45:refnum<k16>)  [unwired: 1 out]
        n124 = String Length(string=w40) -> (length=→"length":i32)
        n125 = UDP Read(connection ID=w45, timeout ms (25000)=100) -> (error out=w33:errorcluster, 3:w35:refnum<k16>)  [unwired: 2 in, 3 out]
        n126 = call <vilib>:"Clear Errors.vi"("error in (no error)"=w33) -> ()  [unwired: 6 in, 1 out]
      }
    }
  }
  n127 = First Call?() -> (First Call?: T/F=w11:bool)
  n128 = case shown="True" w11 {
    frame False {
    }
    frame True {
      n129 = property on="Phase Map" class="IntGraph (strict)"("ZScale.MarkerVals[]"=cluster{dbl, u32}[] [{-3.141, 0}, {0.0, 255}, {3.141, 16777215}] ("Z Scale.Marker Values[]")) -> ()  [unwired: 2 in, 2 out]
    }
  }
  n130 = case shown="False" "Show panel" {
    frame False {
    }
    frame True {
      n131 = property class="VI"("Front Panel.Open"=TRUE ("Front Panel Window:Open")) -> ()  [unwired: 2 in, 2 out]
    }
  }
  n132 = case shown="False" "close" {
    frame False {
    }
    frame True {
      n133 = property class="VI"("Front Panel.Open"=FALSE ("Front Panel Window:Open")) -> ()  [unwired: 2 in, 2 out]
    }
  }
